vi "I2C 4 Channel SPDT Relay Board.vi"() -> ()   [LabVIEW 2020, in "CTI-Scratchpad.lvlib"]
uses:
  CTI-Scratchpad.lvlib
  CTI/Identity.ctl
  CTI/Error Reporting.ctl
  CTI/GPIO Number.ctl
  CTI/I2C Number.ctl
  CTI/Session/Session.lvclass
  CTI-Peripheral/Switching/Grove I2C Switches/4ChannelSPDTRelay.lvclass
  CTI/VisaComms/VisaComms.lvclass
  CTI/CTI.lvlib
panel:
  in  "Load":bool
  out "Switch4LED":bool
  out "Switch3LED":bool
  out "Switch2LED":bool
  out "Switch1LED":bool
  in  "New Address":u8=18 format="%.0x"
  in  "Default Address":u8=17 format="%.0x"
  in  "Stop":bool
  in  "Switch4":bool
  in  "Switch3":bool
  in  "Switch2":bool
  in  "Switch1":bool
  out "loop":i32
  out "Identity":T1
  in  "Grove Connector":enum16{"I2C0", "I2C1"}(ring)
  out "error out":errorcluster
  in  "Port":refnum<visa-resource-name>="COM4"
  # "https://wiki.seeedstudio.com/Grove-4-Channel_SPDT_Relay/"
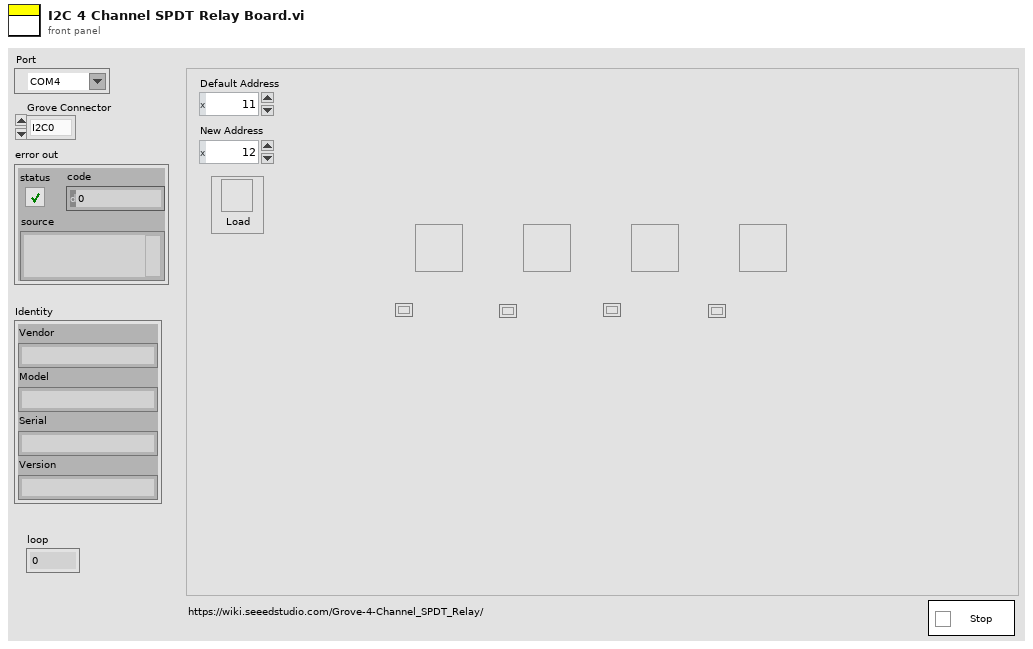
[diagram p1: front panel]
types:
  T1 = typedef "CTI.lvlib/Identity.ctl" = cluster{"Vendor":string, "Model":string, "Serial":string, "Version":string}
  T2 = typedef "CTI.lvlib/Error Reporting.ctl" = enum16{"Minimal", "Moderate", "Full"}
  T3 = typedef "CTI.lvlib/I2C Number.ctl" = i8
  T4 = typedef "CTI.lvlib/GPIO Number.ctl" = i8
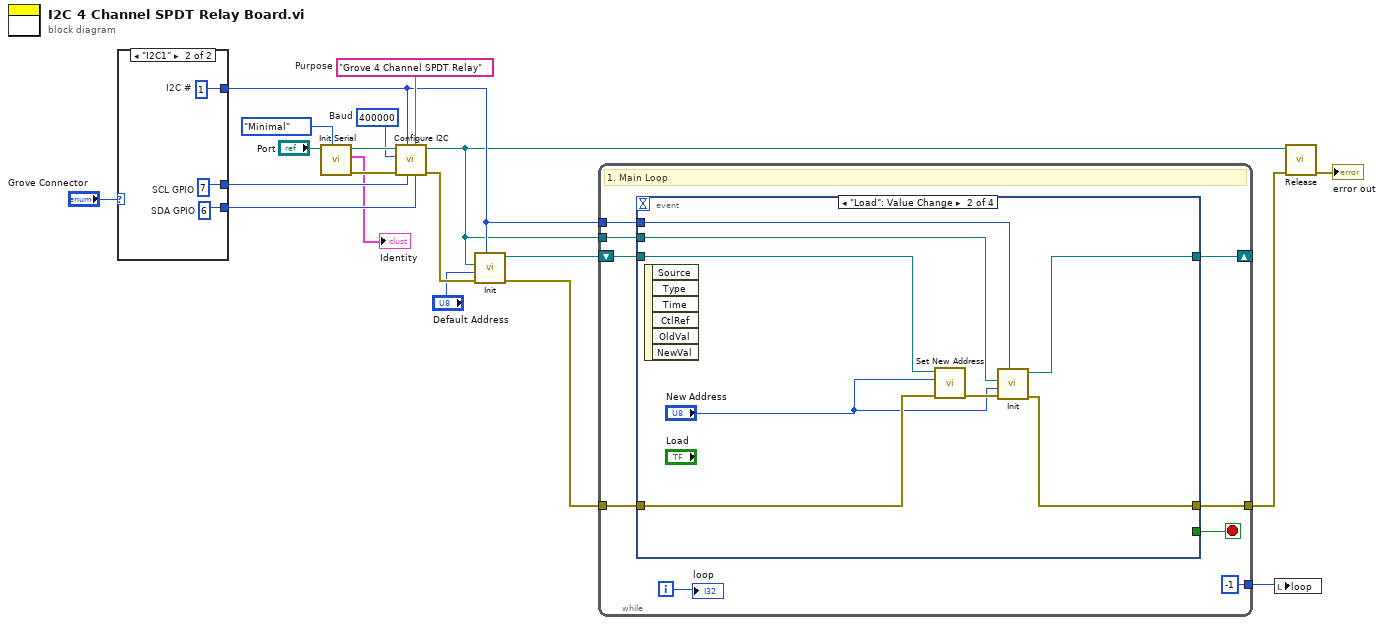
[diagram p0: block diagram]
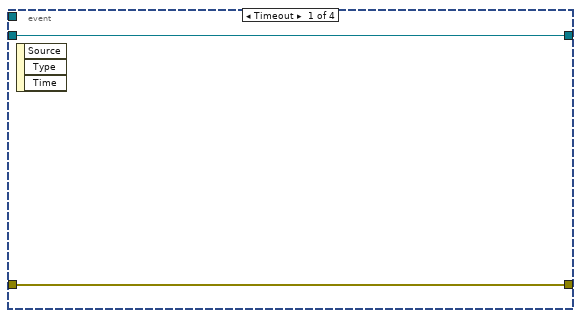
[diagram p2: hidden frame]
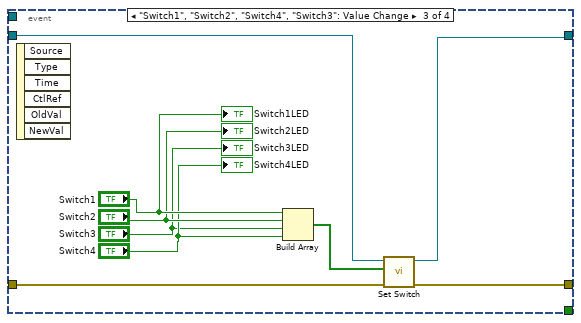
[diagram p3: hidden frame]
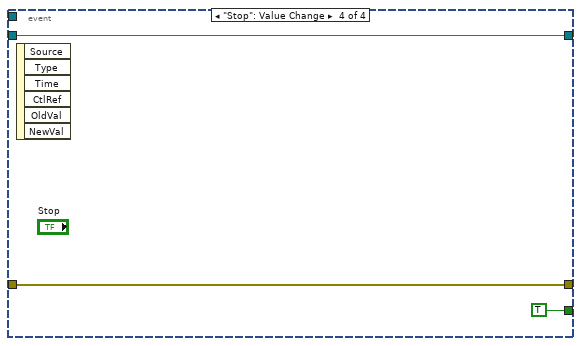
[diagram p4: hidden frame]
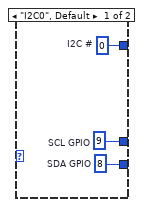
[diagram p5: hidden frame]
diagram:
  w14 = "Grove 4 Channel SPDT Relay"  # Purpose
  w15 = u32 400000  # Baud
  n1 = case shown="\"I2C1\"" "Grove Connector" {
    tunnel: [w22 w25] -> w12
    tunnel: [w21 w24] -> w11
    tunnel: [w20 w23] -> w2
    frame "I2C0", Default {
      w20 = T3 0  # I2C #
      w21 = T4 8  # SDA GPIO
      w22 = T4 9  # SCL GPIO
    }
    frame "I2C1" {
      w23 = T3 1  # I2C #
      w24 = T4 6  # SDA GPIO
      w25 = T4 7  # SCL GPIO
    }
  }
  n2 = call "Init Serial.vi"("Error Checking (Full)"=Error_Reporting."Minimal", "VISA resource name in"="Port") -> ("error out"=w16:errorcluster, "Identity"=→"Identity":T1, "Session"=w17:refnum<class "Session.lvclass">)  [unwired: 7 in]
  n3 = call "Configure I2C.vi"("SDA GPIO"=w11, "Purpose (\"I2C\")"=w14, "SCL GPIO"=w12, "I2C #"=w2, "error in (no error)"=w16, "Baud"=w15, "Session in"=w17) -> ("error out"=w7:errorcluster, "Session out"=w1:refnum<class "Session.lvclass">)  [unwired: 3 in]
  n4 = call "Init.vi"("I2C #"=w2, "error in (no error)"=w7, "Address"="Default Address", "Session In"=w1) -> ("error out"=w5:errorcluster, "4ChannelSPDTRelay Out"=w6:refnum<class "4ChannelSPDTRelay.lvclass">)  [unwired: 6 in]
  n5 = while {
    tunnel: w5 -> [w33]
    tunnel: [w31] -> w9
    tunnel: [-1] -> w4
    shift-right: [w28] -> _
    shift-left: w6 -> [w34]
    tunnel: w2 -> [w27]
    tunnel: w1 -> [w26]
    i -> [w32]
    stop <- w30 stop-if-true
    # "1. Main Loop"
    n6 = event shown="[1] \"Load\": Value Change" {
      selector: _ -> [_ _ _ _]
      dyn-events: _ -> [_ _ _ _]
      timeout: _ -> [_ _ _ _]
      tunnel: w34 -> [w35 w43 w51 w54]
      tunnel: w33 -> [w36 w44 w53 w55]
      tunnel: [w36 w37 w52 w55] -> w31
      tunnel: [_ _ _ TRUE] -> w30
      tunnel: [w35 w41 w50 w54] -> w28
      tunnel: w27 -> [_ w40 _ _]
      tunnel: w26 -> [_ w39 _ _]
      event Timeout {
        n7 = event-data() -> ()  [unwired: 1 in, 3 out]
      }
      event "Load": Value Change {
        n8 = event-data() -> ()  [unwired: 1 in, 6 out]
        n9 = call-dynamic "Set New Address.vi"("error in (no error)"=w44, "New Address"="New Address", "4ChannelSPDTRelay in"=w43) -> ("error out"=w42:errorcluster)  [unwired: 7 in, 1 out]
        n10 = call "Init.vi"("I2C #"=w40, "error in (no error)"=w42, "Address"="New Address", "Session In"=w39) -> ("error out"=w37:errorcluster, "4ChannelSPDTRelay Out"=w41:refnum<class "4ChannelSPDTRelay.lvclass">)  [unwired: 6 in]
      }
      event "Switch1", "Switch2", "Switch4", "Switch3": Value Change {
        n11 = event-data() -> ()  [unwired: 1 in, 6 out]
        n12 = Build Array("Switch1", "Switch2", "Switch3", "Switch4") -> (w49:bool[])
        n13 = call-dynamic "Set Switch.vi"("error in (no error)"=w53, "Switch Settings"=w49, "4ChannelSPDTRelay in"=w51) -> ("error out"=w52:errorcluster, "4ChannelSPDTRelay out"=w50:refnum<class "4ChannelSPDTRelay.lvclass">)  [unwired: 7 in]
        "Switch1LED" <- "Switch1"
        "Switch2LED" <- "Switch2"
        "Switch3LED" <- "Switch3"
        "Switch4LED" <- "Switch4"
      }
      event "Stop": Value Change {
        n14 = event-data() -> ()  [unwired: 1 in, 6 out]
      }
    }
    "loop" <- w32
  }
  n15 = local write "loop"(w4) -> ()
  n16 = call-dynamic "Release.vi"("error in (no error)"=w9, "Session in"=w1) -> ("error out"=→"error out":errorcluster)  [unwired: 9 in]
